vi "ConvertToSec.vi"(0 "raw image data in":dbl[][](array[numeric]) format="%.2f", 1 "reduce pts by factor of":i32=4, 2 "Add Lines":u16=1, 4 "pixels in x":i16=500, 5 "pixels in y":i16=400, 6 "Time between rf pts\nmicros":dbl format="%.2f", 7 "Scan Info":T2 {"delay" format="%.2f"; "pivot distance" format="%.2f"; "sector scan angle" format="%.2f"}, 8 "Abs?":bool=TRUE, 9 "Interp Mode":i32=1, 10 "Smooth factor":i32=3, 11 "use min z value?":bool) -> (15 "raw sector out":dbl[][](array[numeric]) format="%.2f", 18 "Axis scaling Params":T1 {"Y high" format="%.2f"; "Y low" format="%.2f"; "X left" format="%.2f"; "X right" format="%.2f"}, 19 "scales":cluster{"inc x (mm)":dbl, "inc y (mm)":dbl})   [LabVIEW 2022 SP3]
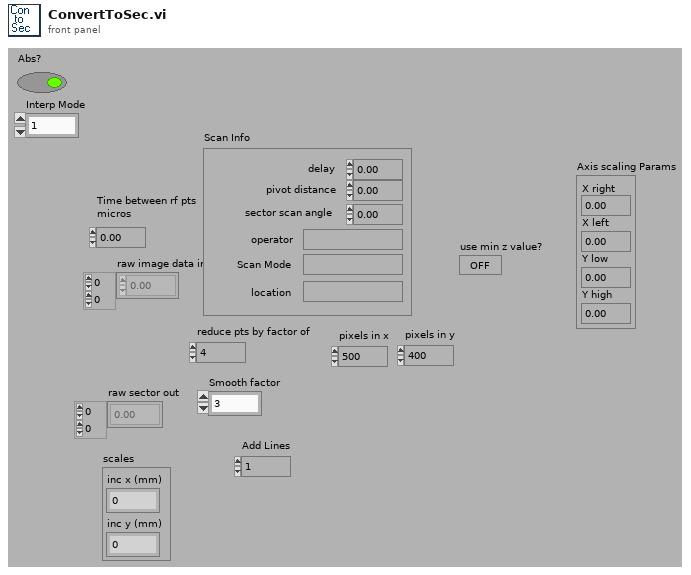
[diagram p1: front panel]
types:
  T1 = cluster{"X right":dbl, "X left":dbl, "Y low":dbl, "Y high":dbl}
  T2 = cluster{"delay":sgl, "pivot distance":sgl, "sector scan angle":sgl, "operator":string, "Scan Mode":string, "location":string}
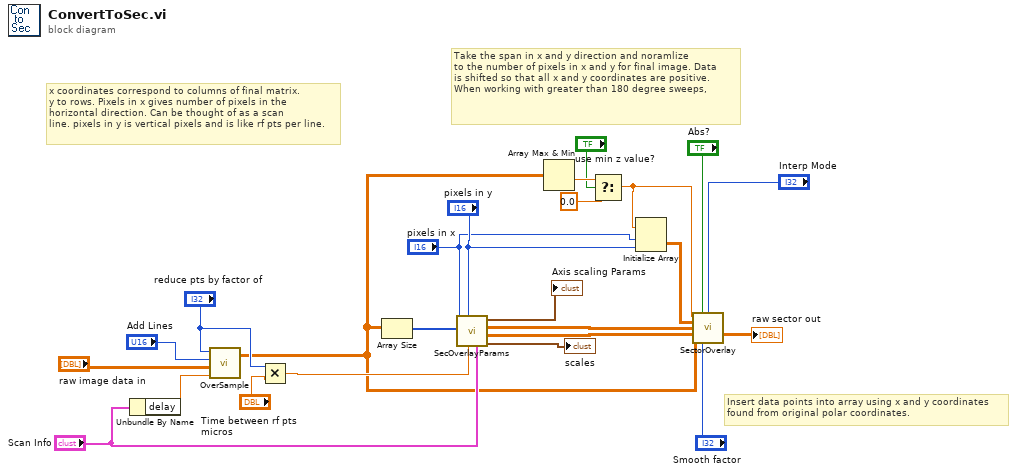
[diagram p0: block diagram]
diagram:
  # "Insert data points into array using x and y coordinates\nfound from original polar coordinates."
  # "Take the span in x and y direction and noramlize\nto the number of pixels in x and y for final image. Data\nis shifted so that all x and y coordinates are positive.\nWhen working with greater than 180 degree sweeps,"
  # "x coordinates correspond to columns of final matrix.\ny to rows. Pixels in x gives number of pixels in the\nhorizontal direction. Can be thought of as a scan\nline. pixels in y is vertical pixels and is like rf pts per line."
  n1 = Unbundle By Name("Scan Info") -> ("delay"=w12:sgl)
  n2 = call "OverSample.vi"("delay"=w12, "raw data in"="raw image data in", "Add Lines"="Add Lines", "reduce RF pts by factor of"="reduce pts by factor of") -> ("reduced data out"=w4:dbl[][])  [unwired: 1 in]
  n3 = Multiply(x="reduce pts by factor of", y="Time between rf pts\nmicros") -> (x*y=w20:dbl)
  n4 = Array Size(array=w4) -> (size(s)=w10:i32[])
  n5 = call "SecOverlayParams.vi"("Scan Info"="Scan Info", "Time between rf pts\nmicros"=w20, "pixels in y"="pixels in y", "Array"=w10, "pixels in x"="pixels in x") -> ("scales"=→"scales":cluster{"inc x (mm)":dbl, "inc y (mm)":dbl}, "y scaled"=w15:dbl[][], "x scaled"=w16:dbl[][], "Axis scaling Params"=→"Axis scaling Params":T1)  [unwired: 3 in]
  n6 = Array Max & Min(array=w4) -> (min value=w24:dbl)  [unwired: 3 out]
  n7 = Select(t=w24, s="use min z value?", f=0.0) -> (s? t:f=w5:dbl)
  n8 = Initialize Array(w5, "pixels in x", "pixels in y") -> (w23:dbl[][])
  n9 = call "SectorOverlay.vi"("Min z"=w5, "Abs?"="Abs?", "Interp Mode"="Interp Mode", "Empty Array"=w23, "x Scaled"=w16, "y Scaled"=w15, "z values"=w4, "Smooth factor"="Smooth factor") -> ("raw sector out"=→"raw sector out":dbl[][])  [unwired: 1 in, 6 out]
